vi "Benchmark Tests.vi"() -> ()   [LabVIEW 2018, in "Colour Lab.lvlib"]
uses:
  Colour Lab.lvlib
panel:
  out "Color":u32(colorbox)
  in  "Lightness(%)":dbl=59.4 format="%#_13g"
  in  "Saturation(%)":dbl=75.8 format="%#_13g"
  in  "Hue(°)":dbl=40.0 format="%#_13g"
  out "Lightness(%)":dbl
  out "Saturation(%)":dbl
  out "Hue(°)":dbl
  out "Time HSL to RGB":dbl
  out "Time RGB to HSL":dbl
  out "Color":u32(colorbox)
  out "Time RGB to Colour Native":dbl
  in  "Blue":u8=73
  in  "Green":u8=177
  in  "Red":u8=230
  out "Color":u32(colorbox)
  out "Time RGB to Colour":dbl
  in  "Blue":u8=73
  in  "Green":u8=177
  in  "Red":u8=230
  out "Blue":u8
  out "Green":u8
  out "Red":u8
  out "Time Colour to RGB Native":dbl
  out "Blue":u8
  out "Green":u8
  out "Red":u8
  out "Time Colour to RGB":dbl
  out "Color":u32(colorbox)
  in  "Value(%)":dbl=90.0 format="%#_13g"
  in  "Saturation(%)":dbl=68.0 format="%#_13g"
  in  "Hue(°)":dbl=40.0 format="%#_13g"
  out "Value(%)":dbl
  out "Saturation(%)":dbl
  out "Hue(°)":dbl
  out "Time HSV to RGB":dbl
  out "Time RGB to HSV":dbl
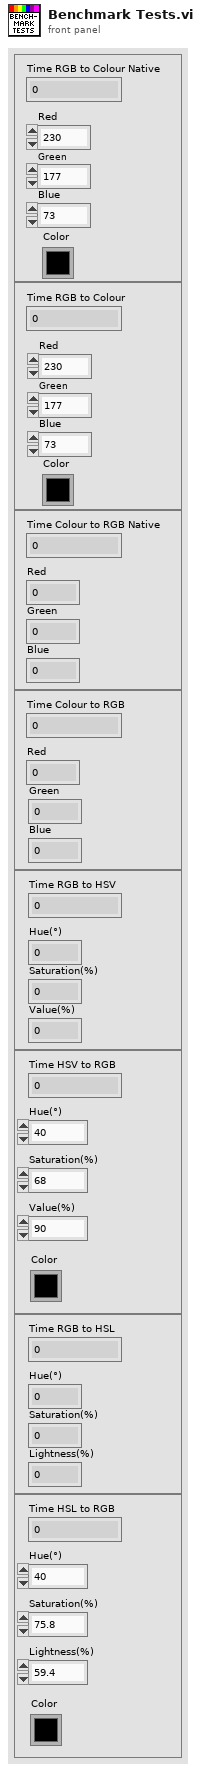
[diagram p1: front panel]
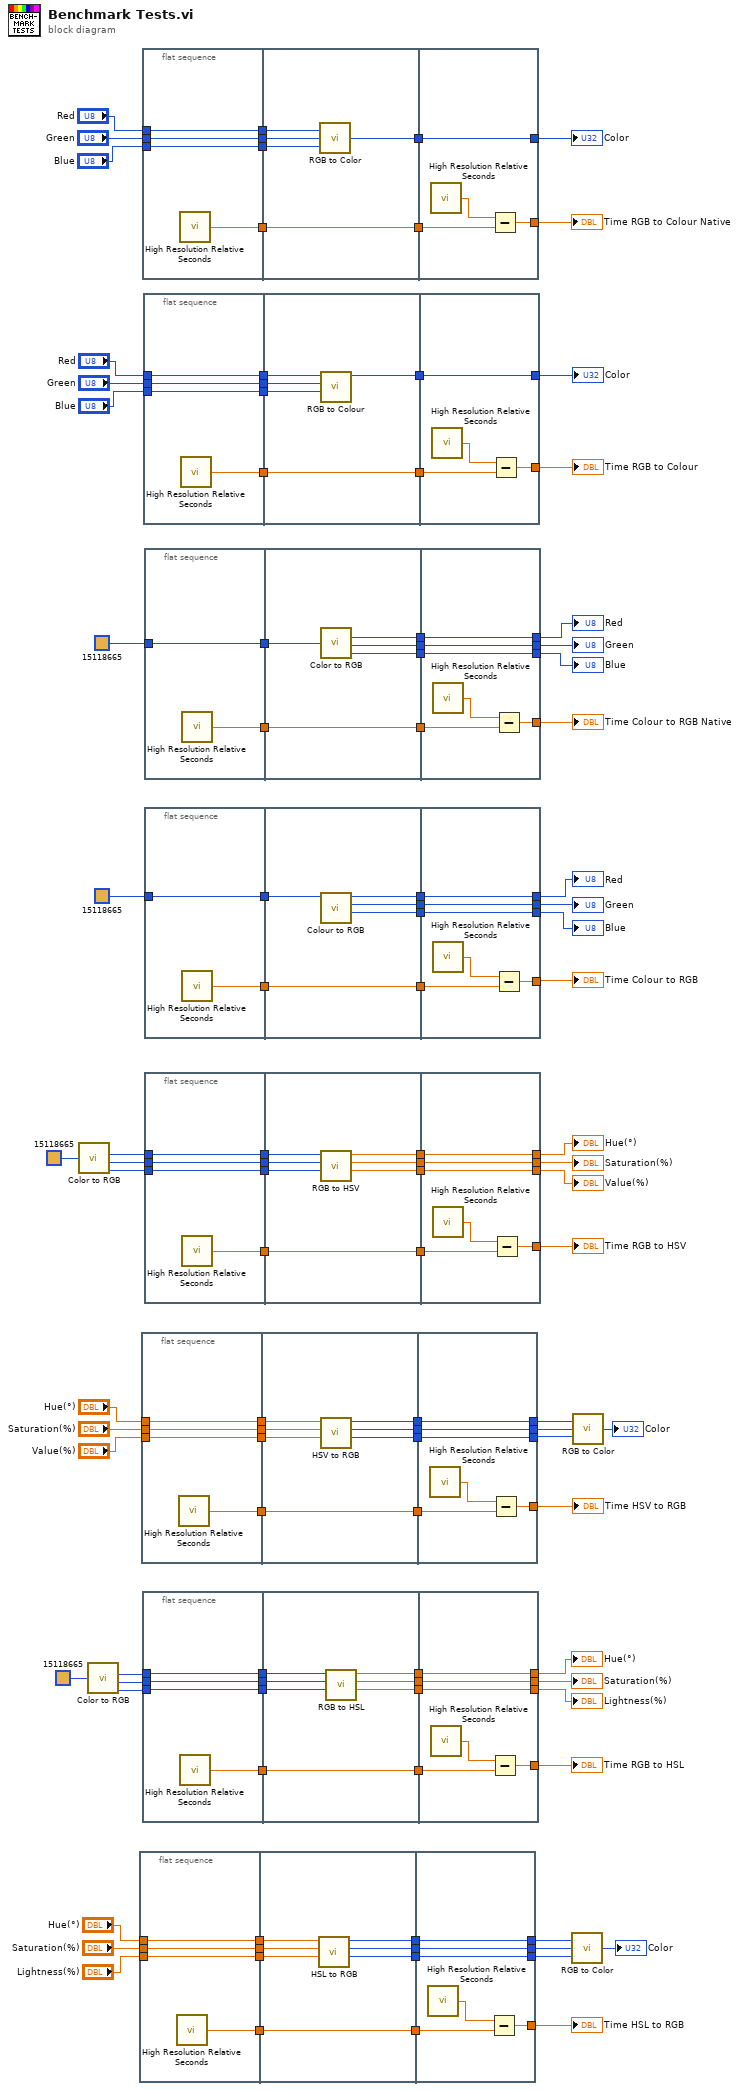
[diagram p0: block diagram]
diagram:
  n1 = call <vilib>:"Color to RGB.vi"("Color"=u32 15118665) -> ("R"=w102:u8, "G"=w101:u8, "B"=w100:u8)  [unwired: 1 out]
  n2 = call <vilib>:"Color to RGB.vi"("Color"=u32 15118665) -> ("R"=w13:u8, "G"=w14:u8, "B"=w15:u8)  [unwired: 1 out]
  n3 = flat-sequence {
    tunnel: [w112] -> w24
    tunnel: "Hue(°)" -> [w111]
    tunnel: [w111] -> w23
    tunnel: "Saturation(%)" -> [w110]
    tunnel: [w110] -> w22
    tunnel: [w109] -> w21
    tunnel: "Lightness(%)" -> [w109]
    tunnel: w24 -> [w119]
    tunnel: [w119] -> w20
    tunnel: w23 -> [w118]
    tunnel: w22 -> [w117]
    tunnel: [w116] -> w19
    tunnel: [w115] -> w18
    tunnel: [w114] -> w17
    tunnel: w21 -> [w113]
    tunnel: w20 -> [w125]
    tunnel: [w123] -> w5
    tunnel: w19 -> [w120]
    tunnel: w18 -> [w121]
    tunnel: w17 -> [w122]
    tunnel: [w122] -> w4
    tunnel: [w121] -> w8
    tunnel: [w120] -> w7
    frame #0 {
      n4 = call <vilib>:"High Resolution Relative Seconds.vi"() -> ("relative seconds"=w112:dbl)
    }
    frame #1 {
      n5 = call "HSL to RGB.vi"("Lightness(%)"=w113, "Saturation(%)"=w117, "Hue(°)"=w118) -> ("Blue"=w114:u8, "Green"=w115:u8, "Red"=w116:u8)  [unwired: 5 in, 1 out]
    }
    frame #2 {
      n6 = call <vilib>:"High Resolution Relative Seconds.vi"() -> ("relative seconds"=w124:dbl)
      n7 = Subtract(x=w124, y=w125) -> (x-y=w123:dbl)
    }
  }
  n8 = flat-sequence {
    tunnel: [w129] -> w105
    tunnel: "Hue(°)" -> [w128]
    tunnel: [w128] -> w88
    tunnel: "Saturation(%)" -> [w127]
    tunnel: [w127] -> w87
    tunnel: [w126] -> w82
    tunnel: "Value(%)" -> [w126]
    tunnel: w105 -> [w136]
    tunnel: [w136] -> w104
    tunnel: w88 -> [w135]
    tunnel: w87 -> [w134]
    tunnel: [w133] -> w85
    tunnel: [w132] -> w84
    tunnel: [w131] -> w83
    tunnel: w82 -> [w130]
    tunnel: w104 -> [w142]
    tunnel: [w140] -> w103
    tunnel: w85 -> [w137]
    tunnel: w84 -> [w138]
    tunnel: w83 -> [w139]
    tunnel: [w139] -> w78
    tunnel: [w138] -> w79
    tunnel: [w137] -> w80
    frame #0 {
      n9 = call <vilib>:"High Resolution Relative Seconds.vi"() -> ("relative seconds"=w129:dbl)
    }
    frame #1 {
      n10 = call "HSV to RGB.vi"("Value(%)"=w130, "Saturation(%)"=w134, "Hue(°)"=w135) -> ("Blue"=w131:u8, "Green"=w132:u8, "Red"=w133:u8)  [unwired: 5 in, 1 out]
    }
    frame #2 {
      n11 = call <vilib>:"High Resolution Relative Seconds.vi"() -> ("relative seconds"=w141:dbl)
      n12 = Subtract(x=w141, y=w142) -> (x-y=w140:dbl)
    }
  }
  n13 = flat-sequence {
    tunnel: [w146] -> w43
    tunnel: "Red" -> [w145]
    tunnel: "Green" -> [w144]
    tunnel: "Blue" -> [w143]
    tunnel: [w145] -> w42
    tunnel: [w144] -> w41
    tunnel: [w143] -> w40
    tunnel: w43 -> [w151]
    tunnel: [w151] -> w39
    tunnel: w42 -> [w150]
    tunnel: w41 -> [w148]
    tunnel: w40 -> [w147]
    tunnel: [w149] -> w38
    tunnel: w39 -> [w155]
    tunnel: [w153] -> w34
    tunnel: w38 -> [w152]
    tunnel: [w152] -> w33
    frame #0 {
      n14 = call <vilib>:"High Resolution Relative Seconds.vi"() -> ("relative seconds"=w146:dbl)
    }
    frame #1 {
      n15 = call <vilib>:"RGB to Color.vi"("B"=w147, "G"=w148, "R"=w150) -> ("Color"=w149:u32)
    }
    frame #2 {
      n16 = call <vilib>:"High Resolution Relative Seconds.vi"() -> ("relative seconds"=w154:dbl)
      n17 = Subtract(x=w154, y=w155) -> (x-y=w153:dbl)
    }
  }
  n18 = flat-sequence {
    tunnel: [w159] -> w32
    tunnel: w13 -> [w158]
    tunnel: w14 -> [w157]
    tunnel: w15 -> [w156]
    tunnel: [w158] -> w31
    tunnel: [w157] -> w30
    tunnel: [w156] -> w29
    tunnel: w32 -> [w166]
    tunnel: [w166] -> w28
    tunnel: w31 -> [w163]
    tunnel: w30 -> [w164]
    tunnel: w29 -> [w165]
    tunnel: [w162] -> w27
    tunnel: [w161] -> w26
    tunnel: [w160] -> w25
    tunnel: w28 -> [w172]
    tunnel: [w170] -> w12
    tunnel: w27 -> [w169]
    tunnel: w26 -> [w168]
    tunnel: w25 -> [w167]
    tunnel: [w169] -> w9
    tunnel: [w168] -> w11
    tunnel: [w167] -> w10
    frame #0 {
      n19 = call <vilib>:"High Resolution Relative Seconds.vi"() -> ("relative seconds"=w159:dbl)
    }
    frame #1 {
      n20 = call "RGB to HSL.vi"("Blue"=w165, "Green"=w164, "Red"=w163) -> ("Lightness(%)"=w162:dbl, "Saturation(%)"=w161:dbl, "Hue(°)"=w160:dbl)  [unwired: 5 in, 1 out]
    }
    frame #2 {
      n21 = call <vilib>:"High Resolution Relative Seconds.vi"() -> ("relative seconds"=w171:dbl)
      n22 = Subtract(x=w171, y=w172) -> (x-y=w170:dbl)
    }
  }
  n23 = flat-sequence {
    tunnel: [w176] -> w54
    tunnel: "Red" -> [w175]
    tunnel: "Green" -> [w174]
    tunnel: "Blue" -> [w173]
    tunnel: [w175] -> w53
    tunnel: [w174] -> w52
    tunnel: [w173] -> w51
    tunnel: w54 -> [w181]
    tunnel: [w181] -> w50
    tunnel: w53 -> [w180]
    tunnel: w52 -> [w179]
    tunnel: w51 -> [w178]
    tunnel: [w177] -> w49
    tunnel: w50 -> [w185]
    tunnel: [w183] -> w45
    tunnel: w49 -> [w182]
    tunnel: [w182] -> w44
    frame #0 {
      n24 = call <vilib>:"High Resolution Relative Seconds.vi"() -> ("relative seconds"=w176:dbl)
    }
    frame #1 {
      n25 = call "RGB to Colour.vi"("Blue"=w178, "Green"=w179, "Red"=w180) -> ("Color"=w177:u32)  [unwired: 7 in, 1 out]
    }
    frame #2 {
      n26 = call <vilib>:"High Resolution Relative Seconds.vi"() -> ("relative seconds"=w184:dbl)
      n27 = Subtract(x=w184, y=w185) -> (x-y=w183:dbl)
    }
  }
  n28 = flat-sequence {
    tunnel: [w187] -> w69
    tunnel: u32 15118665 ("Color") -> [w186]
    tunnel: [w186] -> w68
    tunnel: w69 -> [w192]
    tunnel: [w192] -> w67
    tunnel: [w191] -> w66
    tunnel: [w190] -> w65
    tunnel: [w189] -> w64
    tunnel: w68 -> [w188]
    tunnel: w67 -> [w198]
    tunnel: [w196] -> w58
    tunnel: w66 -> [w193]
    tunnel: w65 -> [w194]
    tunnel: w64 -> [w195]
    tunnel: [w195] -> w55
    tunnel: [w194] -> w57
    tunnel: [w193] -> w56
    frame #0 {
      n29 = call <vilib>:"High Resolution Relative Seconds.vi"() -> ("relative seconds"=w187:dbl)
    }
    frame #1 {
      n30 = call <vilib>:"Color to RGB.vi"("Color"=w188) -> ("R"=w191:u8, "G"=w190:u8, "B"=w189:u8)  [unwired: 1 out]
    }
    frame #2 {
      n31 = call <vilib>:"High Resolution Relative Seconds.vi"() -> ("relative seconds"=w197:dbl)
      n32 = Subtract(x=w197, y=w198) -> (x-y=w196:dbl)
    }
  }
  n33 = flat-sequence {
    tunnel: [w200] -> w76
    tunnel: u32 15118665 ("Color") -> [w199]
    tunnel: [w199] -> w71
    tunnel: w76 -> [w205]
    tunnel: [w205] -> w75
    tunnel: [w202] -> w74
    tunnel: [w203] -> w73
    tunnel: [w204] -> w72
    tunnel: w71 -> [w201]
    tunnel: w75 -> [w211]
    tunnel: [w209] -> w62
    tunnel: w74 -> [w206]
    tunnel: w73 -> [w207]
    tunnel: w72 -> [w208]
    tunnel: [w208] -> w59
    tunnel: [w207] -> w60
    tunnel: [w206] -> w61
    frame #0 {
      n34 = call <vilib>:"High Resolution Relative Seconds.vi"() -> ("relative seconds"=w200:dbl)
    }
    frame #1 {
      n35 = call "Colour to RGB.vi"("Color"=w201) -> ("Blue"=w204:u8, "Green"=w203:u8, "Red"=w202:u8)  [unwired: 6 in, 2 out]
    }
    frame #2 {
      n36 = call <vilib>:"High Resolution Relative Seconds.vi"() -> ("relative seconds"=w210:dbl)
      n37 = Subtract(x=w210, y=w211) -> (x-y=w209:dbl)
    }
  }
  n38 = flat-sequence {
    tunnel: [w215] -> w108
    tunnel: w102 -> [w214]
    tunnel: w101 -> [w213]
    tunnel: w100 -> [w212]
    tunnel: [w214] -> w99
    tunnel: [w213] -> w98
    tunnel: [w212] -> w97
    tunnel: w108 -> [w222]
    tunnel: [w222] -> w107
    tunnel: w99 -> [w221]
    tunnel: w98 -> [w220]
    tunnel: w97 -> [w219]
    tunnel: [w218] -> w96
    tunnel: [w217] -> w95
    tunnel: [w216] -> w94
    tunnel: w107 -> [w228]
    tunnel: [w226] -> w106
    tunnel: w96 -> [w225]
    tunnel: w95 -> [w224]
    tunnel: w94 -> [w223]
    tunnel: [w225] -> w91
    tunnel: [w224] -> w92
    tunnel: [w223] -> w93
    frame #0 {
      n39 = call <vilib>:"High Resolution Relative Seconds.vi"() -> ("relative seconds"=w215:dbl)
    }
    frame #1 {
      n40 = call "RGB to HSV.vi"("Blue"=w219, "Green"=w220, "Red"=w221) -> ("Value(%)"=w218:dbl, "Saturation(%)"=w217:dbl, "Hue(°)"=w216:dbl)  [unwired: 5 in, 1 out]
    }
    frame #2 {
      n41 = call <vilib>:"High Resolution Relative Seconds.vi"() -> ("relative seconds"=w227:dbl)
      n42 = Subtract(x=w227, y=w228) -> (x-y=w226:dbl)
    }
  }
  n43 = call <vilib>:"RGB to Color.vi"("B"=w4, "G"=w8, "R"=w7) -> ("Color"=→"Color":u32)
  n44 = call <vilib>:"RGB to Color.vi"("B"=w78, "G"=w79, "R"=w80) -> ("Color"=→"Color":u32)
  "Time RGB to HSV" <- w106
  "Time HSV to RGB" <- w103
  "Hue(°)" <- w93
  "Saturation(%)" <- w92
  "Value(%)" <- w91
  "Time Colour to RGB" <- w62
  "Red" <- w61
  "Green" <- w60
  "Blue" <- w59
  "Time Colour to RGB Native" <- w58
  "Red" <- w56
  "Green" <- w57
  "Blue" <- w55
  "Time RGB to Colour" <- w45
  "Color" <- w44
  "Time RGB to Colour Native" <- w34
  "Color" <- w33
  "Time RGB to HSL" <- w12
  "Time HSL to RGB" <- w5
  "Hue(°)" <- w10
  "Saturation(%)" <- w11
  "Lightness(%)" <- w9
